vi "HeaderData.vi"   [LabVIEW 2018]
types:
  T1 = enum16{"open", "replace", "create", "open or create", "replace or create", "replace or create with confirmation"}
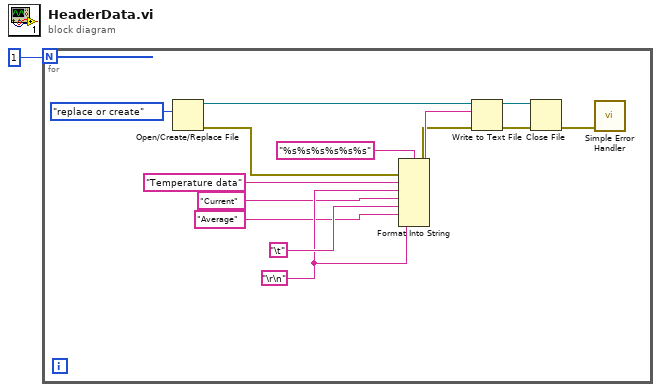
[diagram p0: block diagram]
diagram:
  n1 = for {
    N: 1 ("Numeric") -> [_]
    w13 = "\r\n"
    n2 = Open/Create/Replace File(operation (0:open)=T1."replace or create") -> (refnum out=w4:refnum<file>, error out=w5:errorcluster)  [unwired: 5 in, 1 out]
    n3 = Format Into String(format string="%s%s%s%s%s%s", error in=w5, "Temperature data" ("input 1"), w13, "Current" ("input 3"), "\t", "Average" ("input 5"), w13) -> (resulting string=w7:string, error out=w6:errorcluster)  [unwired: 1 in]
    n4 = Write to Text File(file (use dialog)=w4, text=w7, error in=w6) -> (refnum out=w2:refnum<file>, error out=w8:errorcluster)  [unwired: 1 in, 1 out]
    n5 = Close File(refnum=w2, error in=w8) -> (error out=w9:errorcluster)  [unwired: 1 out]
    n6 = call <vilib>:"Simple Error Handler.vi"("error in (no error)"=w9) -> ()  [unwired: 4 in, 5 out]
  }
